vi "Single String(s) to Stamp.vi"(5 "time string(ms)":string) -> (2 "time stamp(ms)":timestamp format="%<%X\n%x>T")   [LabVIEW 2020]
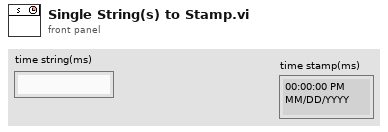
[diagram p1: front panel]
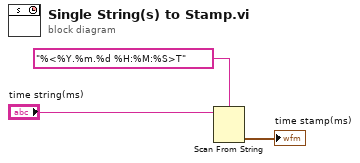
[diagram p0: block diagram]
diagram:
  n1 = Scan From String(format string="%<%Y.%m.%d %H:%M:%S>T", input string="time string(ms)") -> (output 1=→"time stamp(ms)":timestamp)  [unwired: 3 in, 3 out]
